vi "add_Vector3Stamped.vi"(5 "Vector3":cluster{"x":dbl, "y":dbl, "z":dbl}, 6 "Stamp":cluster{"frame_id":string, "reset seq?":bool}, 7 "msg in":string) -> (3 "msg out":string)   [LabVIEW 2012]
doc: "Flattens a vector 3 stamped into a message"
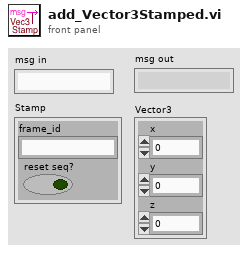
[diagram p1: front panel]
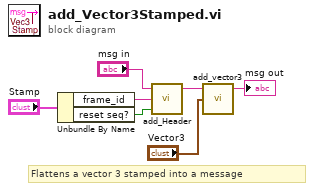
[diagram p0: block diagram]
diagram:
  # "Flattens a vector 3 stamped into a message"
  n1 = Unbundle By Name("Stamp") -> ("frame_id"=w2:string, "reset seq?"=w1:bool)
  n2 = call <userlib>:"add_Header.vi"("reset seq?"=w1, "frame_id"=w2, "msg in"="msg in") -> ("msg out"=w6:string)  [unwired: 2 in]
  n3 = call <userlib>:"add_vector3.vi"("Vector3"="Vector3", "msg in"=w6) -> ("msg out"=→"msg out":string)  [unwired: 3 in]
